vi "Sum Elements in 1D Array.vi"(1 "1D Array In":i32[](array[numeric])) -> (0 "Sum of Elements":i32)   [LabVIEW 2014, in "Initialization and IO Node Scripting.lvlib"]
uses:
  Initialization and IO Node Scripting.lvlib
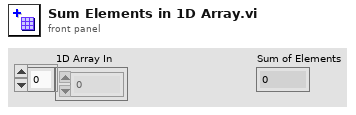
[diagram p1: front panel]
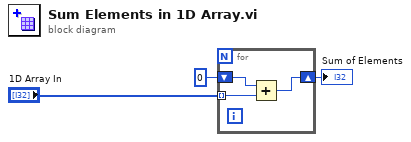
[diagram p0: block diagram]
diagram:
  n1 = for {
    tunnel: "1D Array In" -> [w6] mode=indexing
    shift-right: [w4] -> w2
    shift-left: 0 -> [w5]
    n2 = Add(x=w5, y=w6) -> (x+y=w4:i32)
  }
  "Sum of Elements" <- w2
